vi "Autonomous Independent.vi"() -> ()   [LabVIEW 2012]
doc: "This VI is called when autonomous begins, and will automatically be terminated when autonomous ends. You can carry out timed or sensor driven robot movement independently without needing to return to the caller."
uses:
  Robot Global Data.vi
  <vilib>/Rock Robotics/WPI/RobotDrive/WPI_RobotDriveGetSetRefNum.vi
  <vilib>/Rock Robotics/WPI/Joystick/WPI_JoystickGetSetRefNum.vi
  <vilib>/Rock Robotics/WPI/RobotDrive/WPI_RobotDriveArcadeDrive_Standard(NoSaturation).vi
panel:
  in  "Array of robot movements 2":T1(array[cluster]) {"Y Joystick Value" scale=1.0..-1.0; "X Joystick Value" scale=-1.0..1.0}
  out "Current Movement, for debugging 2":T2 {"Y Joystick Value" scale=1.0..-1.0; "X Joystick Value" scale=-1.0..1.0}
  out "Current Movement, for debugging":T2 {"Y Joystick Value" scale=1.0..-1.0; "X Joystick Value" scale=-1.0..1.0}
  in  "Array of robot movements":T1(array[cluster]) {"Y Joystick Value" scale=1.0..-1.0; "X Joystick Value" scale=-1.0..1.0}
  # "Be sure to right-click and choose Data Operations>>Make Current Value default if you want to save the array values with the VI"
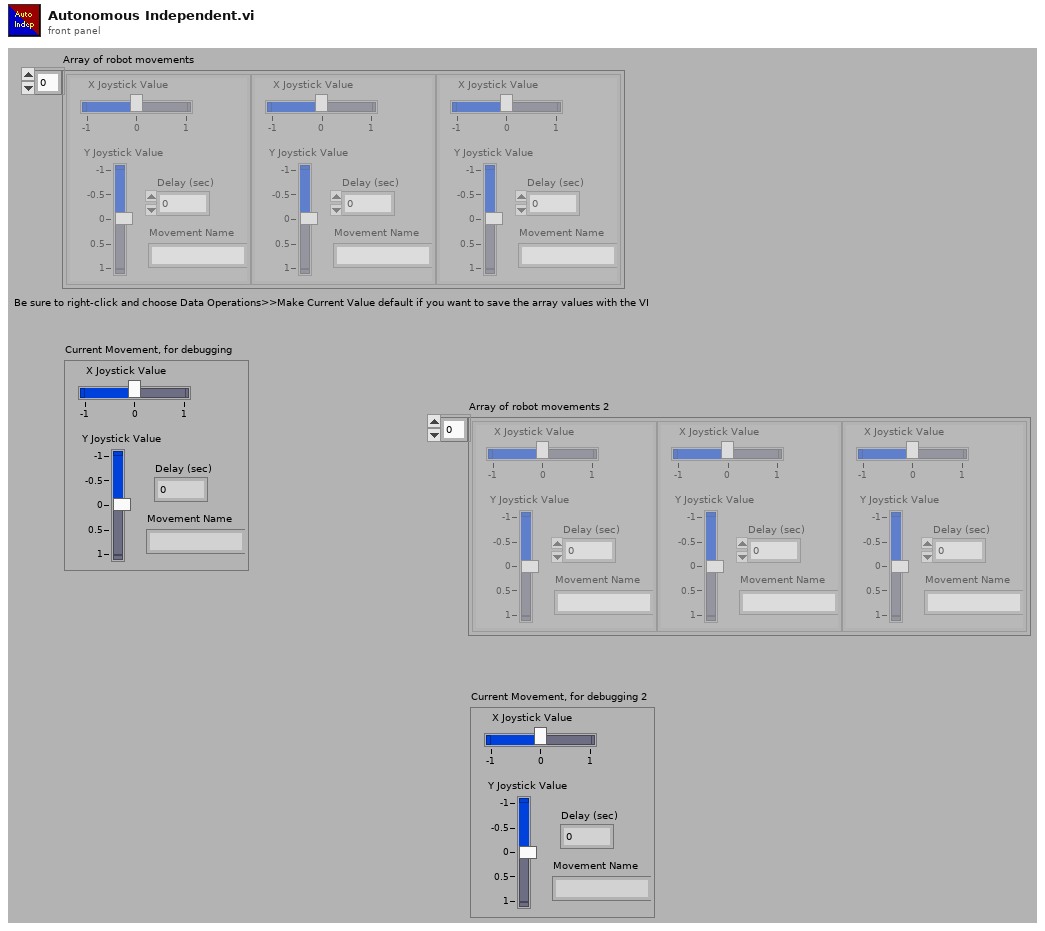
[diagram p1: front panel]
types:
  T1 = cluster{"X Joystick Value":dbl, "Y Joystick Value":dbl, "Delay (sec)":dbl, "Movement Name":string}[]
  T2 = cluster{"X Joystick Value":dbl, "Y Joystick Value":dbl, "Delay (sec)":dbl, "Movement Name":string}
  T3 = typedef "WPI_JoystickDevRef.ctl" = cluster{"Device":T4}
  T4 = typedef "WPI_JoystickDeviceEnum.ctl" = enum16{"USB 1", "USB 2", "USB 3", "USB 4", "Kinect 1", "Kinect 2"}
  T5 = cluster{"axis 1 (x)":dbl, "axis 2 (y)":dbl, "axis 3 (throttle)":dbl, "axis 4":dbl, "axis 5":dbl, "axis 6":dbl}
  T6 = typedef "WPI_RobotDriveDevRef.ctl" = cluster{"DevStatus":errorcluster, "Motors[]":T7[], "Square Inputs":bool, "Max Output":dbl, "Isochronous":bool}
  T7 = typedef "WPI_MotorControlDeviceRef.ctl" = cluster{"DeviceStatus":errorcluster, "Type":enum16{"PWM", "CAN"}, "PWM":cluster{"Digital Module":T8, "PWM Channel":T9, "DeadBand":T10}, "CAN":cluster{"Device Number":u8, "Control Mode":T11, "Semaphore":T12, "Max Vout":dbl}, "Invert":bool, "TransformRef":T13, "InvTransformRef":T13}
  T8 = typedef "FPGA_TypedefDigitalModule.ctl" = enum16{"Digital Module 1", "Digital Module 2"}
  T9 = typedef "FPGA_DIOPWMChannel.ctl" = enum8{"PWM 1", "PWM 2", "PWM 3", "PWM 4", "PWM 5", "PWM 6", "PWM 7", "PWM 8", "PWM 9", "PWM 10", "Invalid"}
  T10 = typedef "WPI_PWMDeadband.ctl" = cluster{"Name":string, "maxPositivePwm":i32, "minPositivePwm":i32, "centerPwm":i32, "maxNegativePwm":i32, "minNegativePwm":i32, "angularRange":u16}
  T11 = typedef "WPI_CANJaguar_ControlMode.ctl" = enum8{"Percent VBus", "Current", "Speed", "Position", "Voltage"}
  T12 = typedef "Semaphore RefNum" = refnum<k1>
  T13 = typedef "WPI_PWMTransform_ConPane.ctl" = refnum<vi>
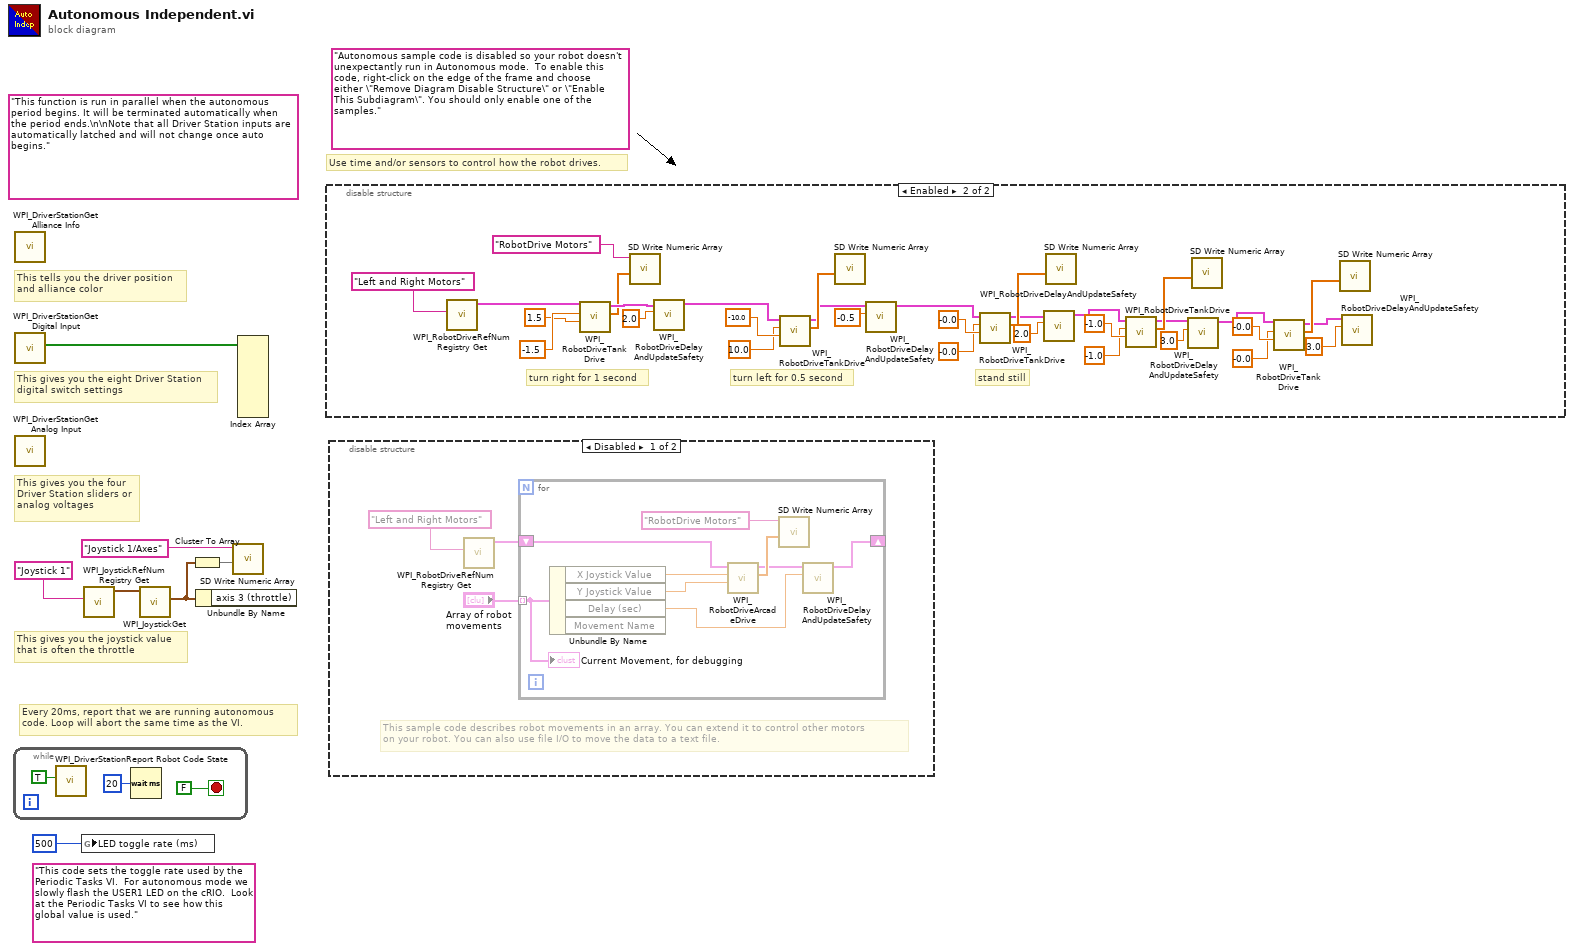
[diagram p0: block diagram]
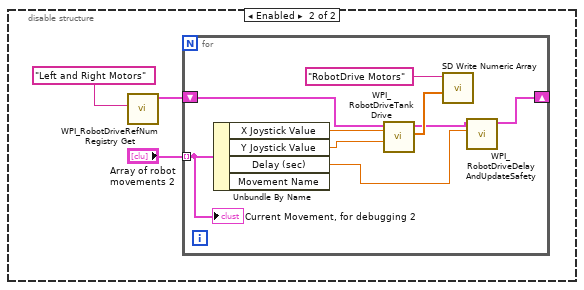
[diagram p2: hidden frame]
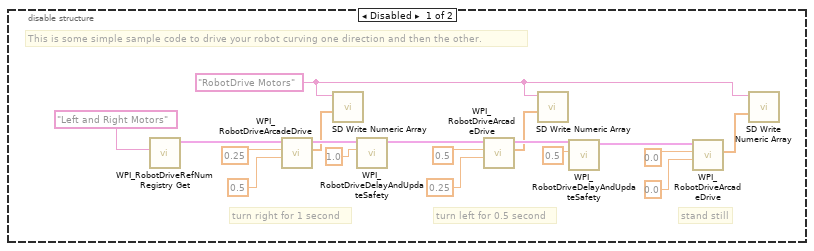
[diagram p3: hidden frame]
diagram:
  (unwired) "This code sets the toggle rate used by the Periodic Tasks VI.  For autonomous mode we slowly flash the USER1 LED on the cRIO.  Look at the Periodic Tasks VI to see how this global value is used."
  (unwired) "Autonomous sample code is disabled so your robot doesn't unexpectantly run in Autonomous mode.  To enable this code, right-click on the edge of the frame and choose either \"Remove Diagram Disable Structure\" or \"Enable This Subdiagram\". You should only enable one of the samples."
  (unwired) "This function is run in parallel when the autonomous period begins. It will be terminated automatically when the period ends.\n\nNote that all Driver Station inputs are automatically latched and will not change once auto begins."
  # "Every 20ms, report that we are running autonomous\ncode. Loop will abort the same time as the VI."
  # "This gives you the joystick value\nthat is often the throttle"
  # "Use time and/or sensors to control how the robot drives."
  # "This tells you the driver position\nand alliance color"
  # "This gives you the eight Driver Station\ndigital switch settings"
  # "This gives you the four\nDriver Station sliders or\nanalog voltages"
  n1 = while {
    stop <- FALSE stop-if-true
    n2 = call <vilib>:"WPI_DriverStationReport Robot Code State.vi"("Autonomous"=TRUE) -> ()  [unwired: 10 in, 1 out]
    n3 = Wait (ms)(milliseconds to wait=u32 20) -> ()  [unwired: 1 out]
  }
  n4 = call <vilib>:"WPI_DriverStationGet Alliance Info.vi"() -> ()  [unwired: 12 out]
  n5 = call <vilib>:"WPI_DriverStationGet Digital Input.vi"() -> ("Driver Station Digital Input (1-8)"=w7:bool[])  [unwired: 11 out]
  n6 = call <vilib>:"WPI_DriverStationGet Analog Input.vi"() -> ()  [unwired: 12 out]
  n7 = global write "Robot Global Data.vi" "LED toggle rate (ms)"(u32 500 ("LED ms toggle rate")) -> ()
  n8 = call <vilib>:"WPI_JoystickRefNum Registry Get.vi"("refnum name"="Joystick 1") -> ("JoystickDevRef"=w5:T3)  [unwired: 1 in, 9 out]
  n9 = call <vilib>:"WPI_JoystickGet.vi"("JoystickDevRef"=w5) -> ("Axes"=w2:T5)  [unwired: 1 in, 5 out]
  n10 = Cluster To Array(cluster=w2) -> (array=w3:dbl[])
  n11 = Unbundle By Name(w2) -> ()  [unwired: 1 out]
  n12 = call <vilib>:"SD Write Numeric Array.vi"("Numeric Array"=w3, "Name"="Joystick 1/Axes") -> ()  [unwired: 8 in, 2 out]
  n13 = Index Array(array=w7) -> ()  [unwired: 8 in, 8 out]
  n14 = disable-structure shown="Enabled" {
    frame Disabled {
      w11 = "RobotDrive Motors" ("Name")
      # "This is some simple sample code to drive your robot curving one direction and then the other."
      # "stand still"
      # "turn left for 0.5 second"
      # "turn right for 1 second"
      n15 = call <vilib>:"WPI_RobotDriveRefNum Registry Get.vi"("refnum name"="Left and Right Motors") -> ("RobotDriveDevRef"=w15:T6)  [unwired: 1 in, 9 out]
      n16 = call-poly <vilib>:"WPI_RobotDriveArcadeDrive.vi"("Y axis value"=0.5 ("X axis value"), "X axis value"=0.25, "RobotDriveDevRef"=w15) -> ("Motor Values"=w14:dbl[], "RobotDriveDevRef"=w22:T6)  [unwired: 1 in, 6 out]
      n17 = call <vilib>:"SD Write Numeric Array.vi"("Numeric Array"=w14, "Name"=w11) -> ()  [unwired: 8 in, 2 out]
      n18 = call <vilib>:"WPI_RobotDriveDelayAndUpdateSafety.vi"("Delay (s)"=1.0, "RobotDriveDevRef"=w22) -> ("RobotDriveDevRef 2"=w21:T6)  [unwired: 8 in, 1 out]
      n19 = call-poly <vilib>:"WPI_RobotDriveArcadeDrive.vi"("Y axis value"=0.25 ("X axis value"), "X axis value"=0.5, "RobotDriveDevRef"=w21) -> ("Motor Values"=w13:dbl[], "RobotDriveDevRef"=w20:T6)  [unwired: 1 in, 6 out]
      n20 = call <vilib>:"SD Write Numeric Array.vi"("Numeric Array"=w13, "Name"=w11) -> ()  [unwired: 8 in, 2 out]
      n21 = call <vilib>:"WPI_RobotDriveDelayAndUpdateSafety.vi"("Delay (s)"=0.5, "RobotDriveDevRef"=w20) -> ("RobotDriveDevRef 2"=w19:T6)  [unwired: 8 in, 1 out]
      n22 = call-poly <vilib>:"WPI_RobotDriveArcadeDrive.vi"("Y axis value"=0.0 ("X axis value"), "X axis value"=0.0, "RobotDriveDevRef"=w19) -> ("Motor Values"=w12:dbl[])  [unwired: 1 in, 7 out]
      n23 = call <vilib>:"SD Write Numeric Array.vi"("Numeric Array"=w12, "Name"=w11) -> ()  [unwired: 8 in, 2 out]
    }
    frame Enabled {
      # "stand still"
      # "turn left for 0.5 second"
      # "turn right for 1 second"
      n24 = call <vilib>:"WPI_RobotDriveRefNum Registry Get.vi"("refnum name"="Left and Right Motors") -> ("RobotDriveDevRef"=w57:T6)  [unwired: 1 in, 9 out]
      n25 = call <vilib>:"WPI_RobotDriveTankDrive.vi"("Right axis value"=1.5 ("X axis value"), "Left axis value"=-1.5 ("X axis value"), "RobotDriveDevRef"=w57) -> ("Motor Values"=w55:dbl[], "RobotDriveDevRef"=w56:T6)  [unwired: 6 in, 1 out]
      n26 = call <vilib>:"SD Write Numeric Array.vi"("Numeric Array"=w55, "Name"="RobotDrive Motors") -> ()  [unwired: 8 in, 2 out]
      n27 = call <vilib>:"WPI_RobotDriveDelayAndUpdateSafety.vi"("Delay (s)"=2.0, "RobotDriveDevRef"=w56) -> ("RobotDriveDevRef 2"=w49:T6)  [unwired: 8 in, 1 out]
      n28 = call <vilib>:"WPI_RobotDriveTankDrive.vi"("Right axis value"=-10.0 ("X axis value"), "Left axis value"=10.0 ("X axis value"), "RobotDriveDevRef"=w49) -> ("Motor Values"=w50:dbl[], "RobotDriveDevRef"=w48:T6)  [unwired: 6 in, 1 out]
      n29 = call <vilib>:"SD Write Numeric Array.vi"("Numeric Array"=w50) -> ()  [unwired: 9 in, 2 out]
      n30 = call <vilib>:"WPI_RobotDriveDelayAndUpdateSafety.vi"("Delay (s)"=-0.5, "RobotDriveDevRef"=w48) -> ("RobotDriveDevRef 2"=w45:T6)  [unwired: 8 in, 1 out]
      n31 = call <vilib>:"WPI_RobotDriveTankDrive.vi"("Right axis value"=-0.0 ("X axis value"), "Left axis value"=-0.0 ("X axis value"), "RobotDriveDevRef"=w45) -> ("Motor Values"=w44:dbl[], "RobotDriveDevRef"=w33:T6)  [unwired: 6 in, 1 out]
      n32 = call <vilib>:"WPI_RobotDriveDelayAndUpdateSafety.vi"("Delay (s)"=2.0, "RobotDriveDevRef"=w33) -> ("RobotDriveDevRef 2"=w32:T6)  [unwired: 8 in, 1 out]
      n33 = call <vilib>:"SD Write Numeric Array.vi"("Numeric Array"=w44) -> ()  [unwired: 9 in, 2 out]
      n34 = call <vilib>:"WPI_RobotDriveTankDrive.vi"("Right axis value"=-1.0 ("X axis value"), "Left axis value"=-1.0 ("X axis value"), "RobotDriveDevRef"=w32) -> ("Motor Values"=w41:dbl[], "RobotDriveDevRef"=w31:T6)  [unwired: 6 in, 1 out]
      n35 = call <vilib>:"WPI_RobotDriveDelayAndUpdateSafety.vi"("Delay (s)"=3.0, "RobotDriveDevRef"=w31) -> ("RobotDriveDevRef 2"=w30:T6)  [unwired: 8 in, 1 out]
      n36 = call <vilib>:"SD Write Numeric Array.vi"("Numeric Array"=w41) -> ()  [unwired: 9 in, 2 out]
      n37 = call <vilib>:"WPI_RobotDriveTankDrive.vi"("Right axis value"=-0.0 ("X axis value"), "Left axis value"=-0.0 ("X axis value"), "RobotDriveDevRef"=w30) -> ("Motor Values"=w38:dbl[], "RobotDriveDevRef"=w29:T6)  [unwired: 6 in, 1 out]
      n38 = call <vilib>:"SD Write Numeric Array.vi"("Numeric Array"=w38) -> ()  [unwired: 9 in, 2 out]
      n39 = call <vilib>:"WPI_RobotDriveDelayAndUpdateSafety.vi"("Delay (s)"=3.0, "RobotDriveDevRef"=w29) -> ()  [unwired: 8 in, 2 out]
    }
  }
  n40 = disable-structure shown="Disabled" {
    frame Disabled {
      # "This sample code describes robot movements in an array. You can extend it to control other motors\non your robot. You can also use file I/O to move the data to a text file."
      n41 = call <vilib>:"WPI_RobotDriveRefNum Registry Get.vi"("refnum name"="Left and Right Motors") -> ("RobotDriveDevRef"=w62:T6)  [unwired: 1 in, 9 out]
      n42 = for {
        shift-right: [w68] -> _
        shift-left: w62 -> [w69]
        tunnel: "Array of robot movements" -> [w64] mode=indexing
        n43 = Unbundle By Name(w64) -> ("X Joystick Value"=w67:dbl, "Y Joystick Value"=w66:dbl, "Delay (sec)"=w65:dbl)  [unwired: 1 out]
        n44 = call-poly <vilib>:"WPI_RobotDriveArcadeDrive.vi"("Y axis value"=w66, "X axis value"=w67, "RobotDriveDevRef"=w69) -> ("Motor Values"=w71:dbl[], "RobotDriveDevRef"=w70:T6)  [unwired: 1 in, 6 out]
        n45 = call <vilib>:"SD Write Numeric Array.vi"("Numeric Array"=w71, "Name"="RobotDrive Motors") -> ()  [unwired: 8 in, 2 out]
        n46 = call <vilib>:"WPI_RobotDriveDelayAndUpdateSafety.vi"("Delay (s)"=w65, "RobotDriveDevRef"=w70) -> ("RobotDriveDevRef 2"=w68:T6)  [unwired: 8 in, 1 out]
        "Current Movement, for debugging" <- w64
      }
    }
    frame Enabled {
      n47 = call <vilib>:"WPI_RobotDriveRefNum Registry Get.vi"("refnum name"="Left and Right Motors") -> ("RobotDriveDevRef"=w74:T6)  [unwired: 1 in, 9 out]
      n48 = for {
        shift-right: [w83] -> _
        shift-left: w74 -> [w76]
        tunnel: "Array of robot movements 2" -> [w81] mode=indexing
        n49 = Unbundle By Name(w81) -> ("X Joystick Value"=w80:dbl, "Y Joystick Value"=w79:dbl, "Delay (sec)"=w82:dbl)  [unwired: 1 out]
        n50 = call <vilib>:"WPI_RobotDriveTankDrive.vi"("Right axis value"=w79, "Left axis value"=w80, "RobotDriveDevRef"=w76) -> ("Motor Values"=w78:dbl[], "RobotDriveDevRef"=w77:T6)  [unwired: 6 in, 1 out]
        n51 = call <vilib>:"SD Write Numeric Array.vi"("Numeric Array"=w78, "Name"="RobotDrive Motors") -> ()  [unwired: 8 in, 2 out]
        n52 = call <vilib>:"WPI_RobotDriveDelayAndUpdateSafety.vi"("Delay (s)"=w82, "RobotDriveDevRef"=w77) -> ("RobotDriveDevRef 2"=w83:T6)  [unwired: 8 in, 1 out]
        "Current Movement, for debugging 2" <- w81
      }
    }
  }
